vi "Modbus test.vi"() -> ()   [LabVIEW 2022 SP3]
uses:
  Controls/Driver_States.ctl
  Modbus Test/Controls/Options.ctl
  Modbus Test/Controls/TestData.ctl
panel:
  in  "ON/OFF":bool[](array[boolean])
  in  "Write Coil":bool
  in  "Coil Address":u16[](array[numeric]) format="%.0x"
  in  "Write Register\n Address":u16[](array[numeric]) format="%.0x"
  in  "Register to write":u16[](array[numeric]) format="%.0x"
  out "Object ID":string
  in  "Port":u16
  in  "Device Address":string
  in  "Exit":bool
  in  "Write Register":bool
  in  "Read Register":bool
  in  "Initialize":bool
  in  "Address":u16[](array[numeric]) format="%.0x"
  in  "Error in":errorcluster
  out "Error out":errorcluster
  out "register values":u16[](array[numeric])
  in  "No Of Inputs":u16
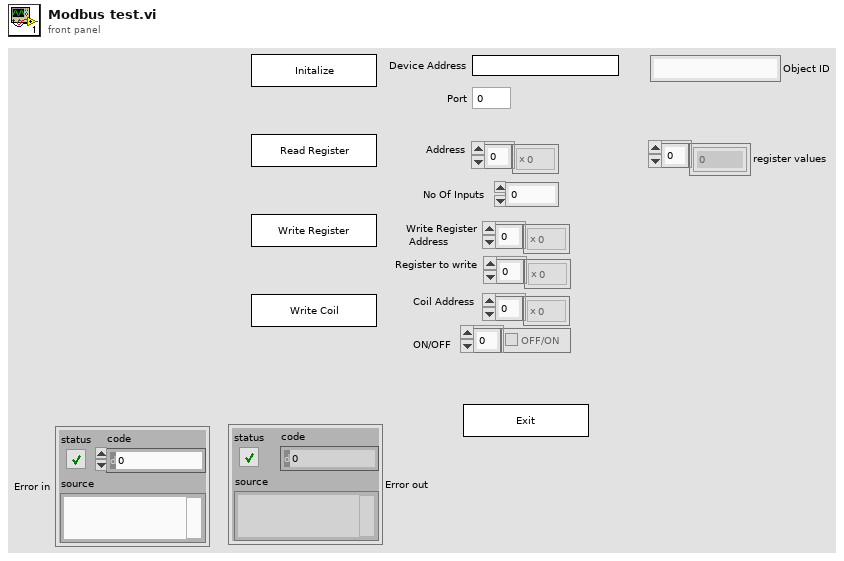
[diagram p1: front panel]
types:
  T1 = typedef "Options.ctl" = enum16{"Poll", "Initialise", "Read Register", "Write Register", "Write Coil", "Error", "Exit"}
  T2 = typedef "TestData.ctl" = cluster{"Address":string, "port (502)":u16, "Starting Address":u16[], "Input Registers to write":u16[], "No Of Inputs":u16, "Coils to write":bool[]}
  T3 = typedef "Driver_States.ctl" = enum16{"Poll", "Initialize", "Read Coil", "Read Multiple Coil", "Read Holding Register", "Read Multiple Holding Registers", "Read Multiple Register", "Write Single Coil", "Write Multiple Coils", "Write Multiple Register", "Read/Write", "Error", "Shutdown", "Exit"}
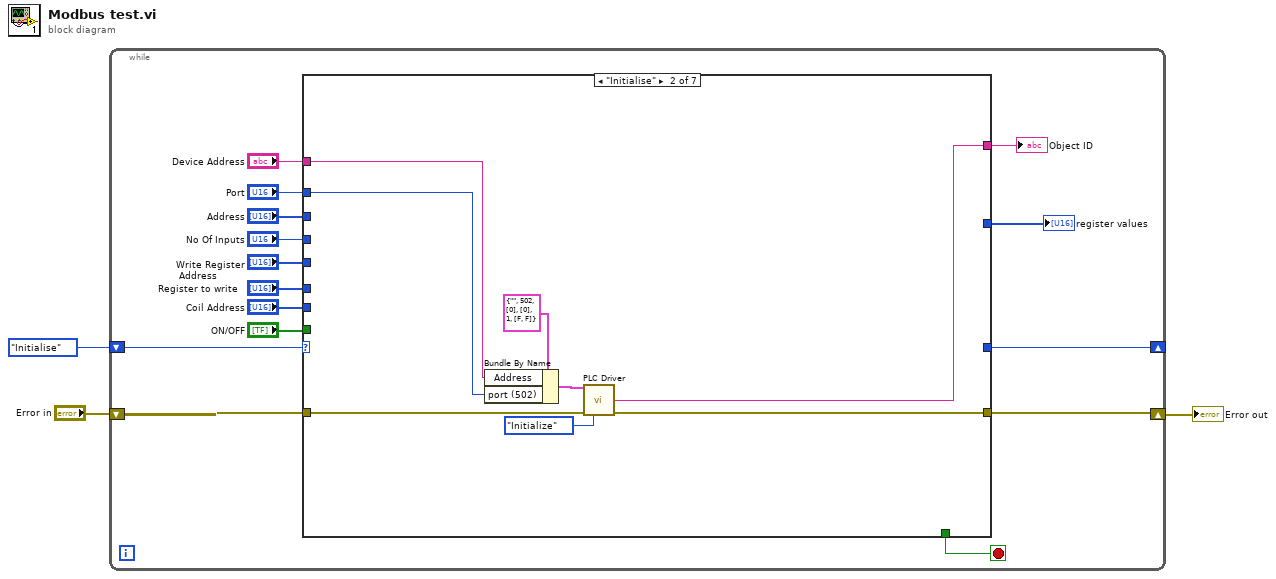
[diagram p0: block diagram]
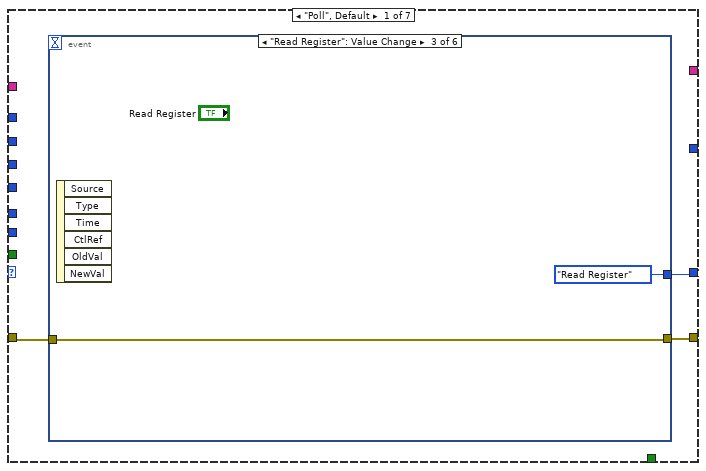
[diagram p2: hidden frame]
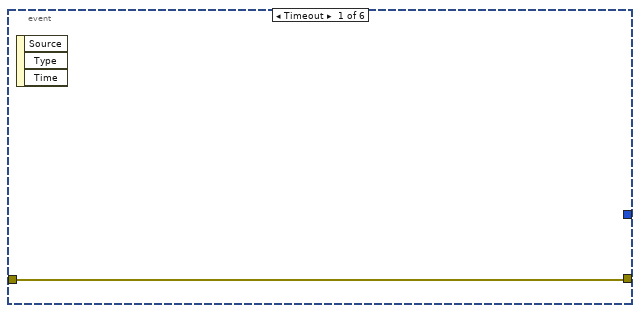
[diagram p3: hidden frame]
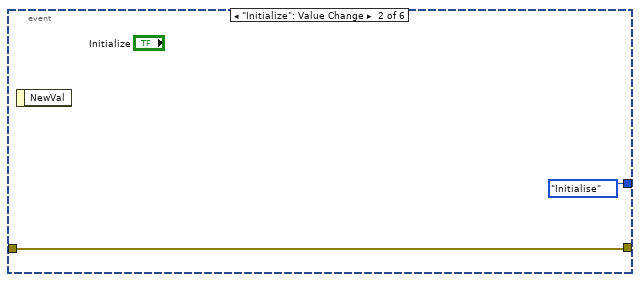
[diagram p4: hidden frame]
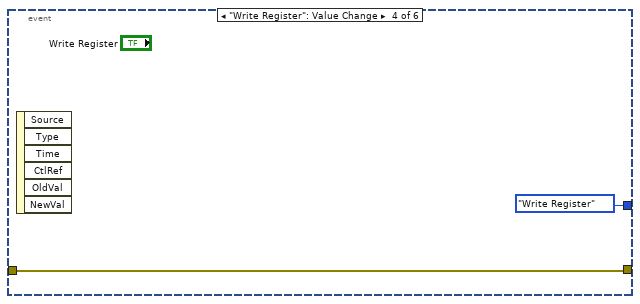
[diagram p5: hidden frame]
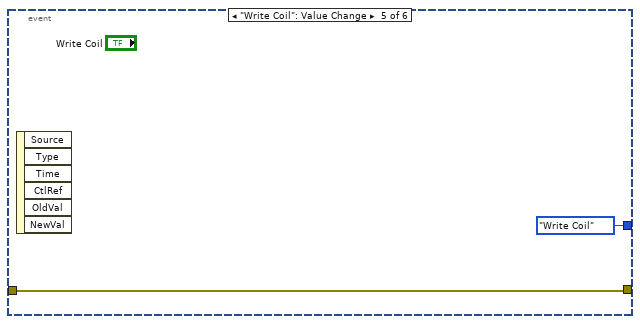
[diagram p6: hidden frame]
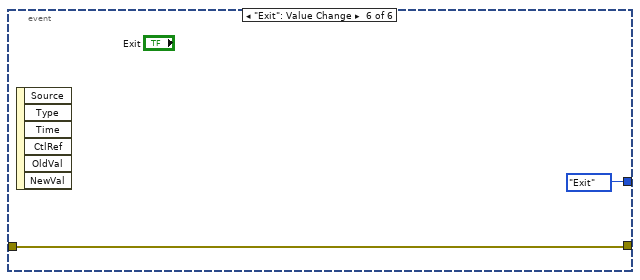
[diagram p7: hidden frame]
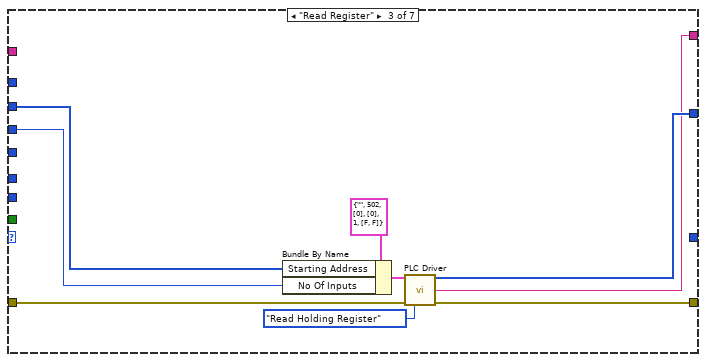
[diagram p8: hidden frame]
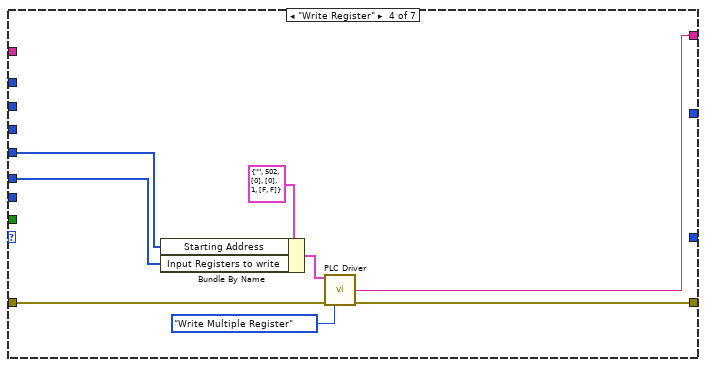
[diagram p9: hidden frame]
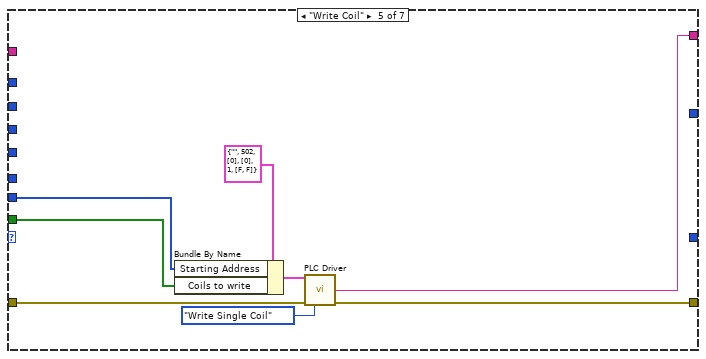
[diagram p10: hidden frame]
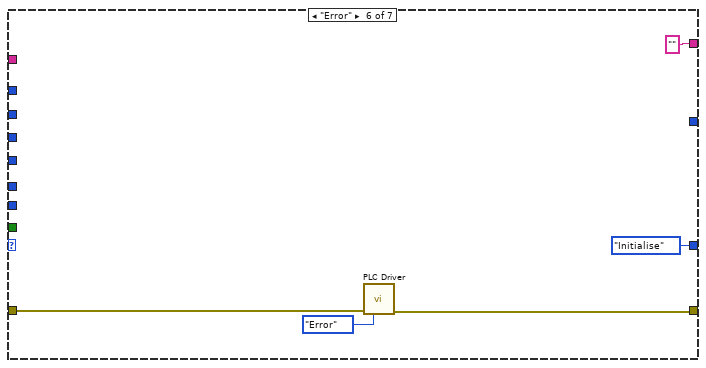
[diagram p11: hidden frame]
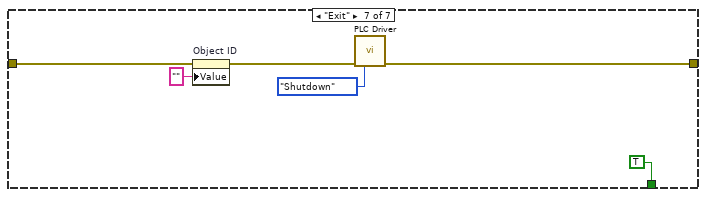
[diagram p12: hidden frame]
diagram:
  n1 = while {
    shift-right: [w17] -> _
    shift-left: Options."Initialise" ("Options") -> [w18]
    shift-right: [w15] -> w1
    shift-left: "Error in" -> [w16]
    stop <- w8 stop-if-true
    n2 = case shown="\"Initialise\"" w18 {
      tunnel: [w21 _ _ _ _ Options."Initialise" ("Options") _] -> w17
      tunnel: [_ _ _ _ _ _ TRUE] -> w8
      tunnel: w16 -> [w20 w40 w45 w54 w64 w69 w73]
      tunnel: [w19 w39 w46 w52 w65 w70 w76] -> w15
      tunnel: "Device Address" -> [_ w36 _ _ _ _ _]
      tunnel: "Port" -> [_ w35 _ _ _ _ _]
      tunnel: [_ w33 w41 w50 w58 "" ("Value") _] -> w4
      tunnel: [_ _ w44 _ _ _ _] -> w12
      tunnel: "Address" -> [_ _ w43 _ _ _ _]
      tunnel: "No Of Inputs" -> [_ _ w42 _ _ _ _]
      tunnel: "Register to write" -> [_ _ _ w55 _ _ _]
      tunnel: "Write Register\n Address" -> [_ _ _ w51 _ _ _]
      tunnel: "Coil Address" -> [_ _ _ _ w60 _ _]
      tunnel: "ON/OFF" -> [_ _ _ _ w59 _ _]
      frame "Poll", Default {
        n3 = event shown="[2] \"Read Register\": Value Change" {
          selector: _ -> [_ _ _ _ _ _]
          dyn-events: _ -> [_ _ _ _ _ _]
          timeout: _ -> [_ _ _ _ _ _]
          tunnel: [_ Options."Initialise" ("Options") Options."Read Register" ("Options") Options."Write Register" ("Options") Options."Write Coil" ("Options") Options."Exit" ("Options")] -> w21
          tunnel: [w22 w23 w25 w27 w30 w31] -> w19
          tunnel: w20 -> [w22 w23 w25 w27 w30 w31]
          event Timeout {
            n4 = event-data() -> ()  [unwired: 1 in, 3 out]
          }
          event "Initialize": Value Change {
            n5 = event-data() -> ()  [unwired: 1 in, 1 out]
          }
          event "Read Register": Value Change {
            n6 = event-data() -> ()  [unwired: 1 in, 6 out]
          }
          event "Write Register": Value Change {
            n7 = event-data() -> ()  [unwired: 1 in, 6 out]
          }
          event "Write Coil": Value Change {
            n8 = event-data() -> ()  [unwired: 1 in, 6 out]
          }
          event "Exit": Value Change {
            n9 = event-data() -> ()  [unwired: 1 in, 6 out]
          }
        }
      }
      frame "Initialise" {
        n10 = Bundle By Name(cluster=T2 {"Address"="", "port (502)"=502, "Starting Address"=[0], "Input Registers to write"=[0], "No Of Inputs"=1, "Coils to write"=[FALSE, FALSE]} ("Input Cluster"), "Address"=w36, "port (502)"=w35) -> (w37:T2)
        n11 = call "PLC Driver.vi"("Data Cluster"=w37, "Error in"=w40, "Options"=Driver_States."Initialize") -> ("Object ID"=w33:string, "Error out"=w39:errorcluster)  [unwired: 9 in, 2 out]
      }
      frame "Read Register" {
        n12 = Bundle By Name(cluster=T2 {"Address"="", "port (502)"=502, "Starting Address"=[0], "Input Registers to write"=[0], "No Of Inputs"=1, "Coils to write"=[FALSE, FALSE]} ("Input Cluster"), "Starting Address"=w43, "No Of Inputs"=w42) -> (w49:T2)
        n13 = call "PLC Driver.vi"("Data Cluster"=w49, "Error in"=w45, "Options"=Driver_States."Read Holding Register") -> ("register values"=w44:u16[], "Object ID"=w41:string, "Error out"=w46:errorcluster)  [unwired: 9 in, 1 out]
      }
      frame "Write Register" {
        n14 = Bundle By Name(cluster=T2 {"Address"="", "port (502)"=502, "Starting Address"=[0], "Input Registers to write"=[0], "No Of Inputs"=1, "Coils to write"=[FALSE, FALSE]} ("Input Cluster"), "Starting Address"=w51, "Input Registers to write"=w55) -> (w57:T2)
        n15 = call "PLC Driver.vi"("Data Cluster"=w57, "Error in"=w54, "Options"=Driver_States."Write Multiple Register") -> ("Object ID"=w50:string, "Error out"=w52:errorcluster)  [unwired: 9 in, 2 out]
      }
      frame "Write Coil" {
        n16 = Bundle By Name(cluster=T2 {"Address"="", "port (502)"=502, "Starting Address"=[0], "Input Registers to write"=[0], "No Of Inputs"=1, "Coils to write"=[FALSE, FALSE]} ("Input Cluster"), "Starting Address"=w60, "Coils to write"=w59) -> (w62:T2)
        n17 = call "PLC Driver.vi"("Data Cluster"=w62, "Error in"=w64, "Options"=Driver_States."Write Single Coil") -> ("Object ID"=w58:string, "Error out"=w65:errorcluster)  [unwired: 9 in, 2 out]
      }
      frame "Error" {
        n18 = call "PLC Driver.vi"("Error in"=w69, "Options"=Driver_States."Error") -> ("Error out"=w70:errorcluster)  [unwired: 10 in, 3 out]
      }
      frame "Exit" {
        n19 = property on="Object ID" class="Str"(error in=w73, "Value"="" ("Object ID")) -> (error out=w72:errorcluster)  [unwired: 1 in, 1 out]
        n20 = call "PLC Driver.vi"("Error in"=w72, "Options"=Driver_States."Shutdown") -> ("Error out"=w76:errorcluster)  [unwired: 10 in, 3 out]
      }
    }
    "register values" <- w12
    "Object ID" <- w4
  }
  "Error out" <- w1
